vi "test - load and unload.vi"(8 "error in (no error)":errorcluster, 11 "TestCase in":refnum<class "csm-ini-variable-addon.lvclass">) -> (0 "error out":errorcluster, 3 "TestCase out":refnum<class "csm-ini-variable-addon.lvclass">)   [LabVIEW 2017, in "csm-ini-variable-addon.lvclass"]
uses:
  csm-ini-variable-addon.lvclass
  07da2d0f-c6b1-41ab-9bdc-e75734193e5e.vi
  7f30f570-6f21-4deb-b8b3-798b22e0b6ad.vi
  07da2d0f-c6b1-41ab-9bdc-e75734193e5e.vi/b09b9099-6be0-413b-8afc-4908471460c3.vi
  INI-Static-Variable-Support/_Support/FlagInstance-CSMINIVariable.vi
  7f30f570-6f21-4deb-b8b3-798b22e0b6ad.vi/b09b9099-6be0-413b-8afc-4908471460c3.vi
  <userlib>/_NEVSTOP/Communicable State Machine(CSM)/_Support/ChangeFlag/ChangeFlag-Read.vi
  <userlib>/_NEVSTOP/Communicable State Machine(CSM)/_Support/ChangeFlag/ChangeFlagDB.vi
  <vilib>/Utility/Data Type/Get Type Information.vi
  <userlib>/_NEVSTOP/Communicable State Machine(CSM)/addons/API-String-Arugments-Support/_Support/Data To SingleElementsArray_csm.vi
  INI-Static-Variable-Support/_Support/Parse Used Session and Name.vi
  <userlib>/_NEVSTOP/Communicable State Machine(CSM)/addons/API-String-Arugments-Support/_Support/Data To API String Arguments.vi
  INI-Static-Variable-Support/_Support/INI-FGV(lvlibp).vi
  INI-Static-Variable-Support/_Support/Populate String with INI Variable.vi
  <userlib>/_NEVSTOP/Communicable State Machine(CSM)/addons/API-String-Arugments-Support/_Support/Convert API String Arguments to Data(variant).vi
  <userlib>/_NEVSTOP/Communicable State Machine(CSM)/addons/API-String-Arugments-Support/_Support/SingleElementsArray To Data_csm.vi
  <vilib>/addons/_JKI Toolkits/VI Tester/TestCase.llb/TestCase.lvclass
  INI-Static-Variable-Support/INI-Static-Variable-Support.lvlib
  <userlib>/_NEVSTOP/Communicable State Machine(CSM)/addons/API-String-Arugments-Support/API String Arguments Support.lvlib
  C:/Program Files (x86)/National Instruments/LabVIEW 2017/vi.lib/addons/_JKI Toolkits/VI Tester/TestCase.llb/TestCase.lvclass
panel:
  out "String out":string
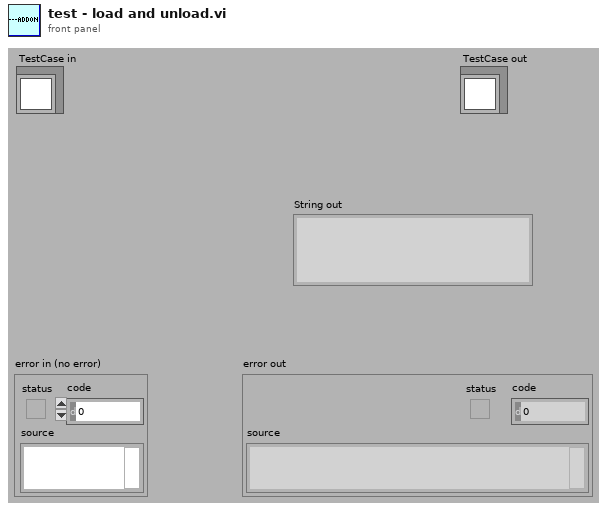
[diagram p1: front panel]
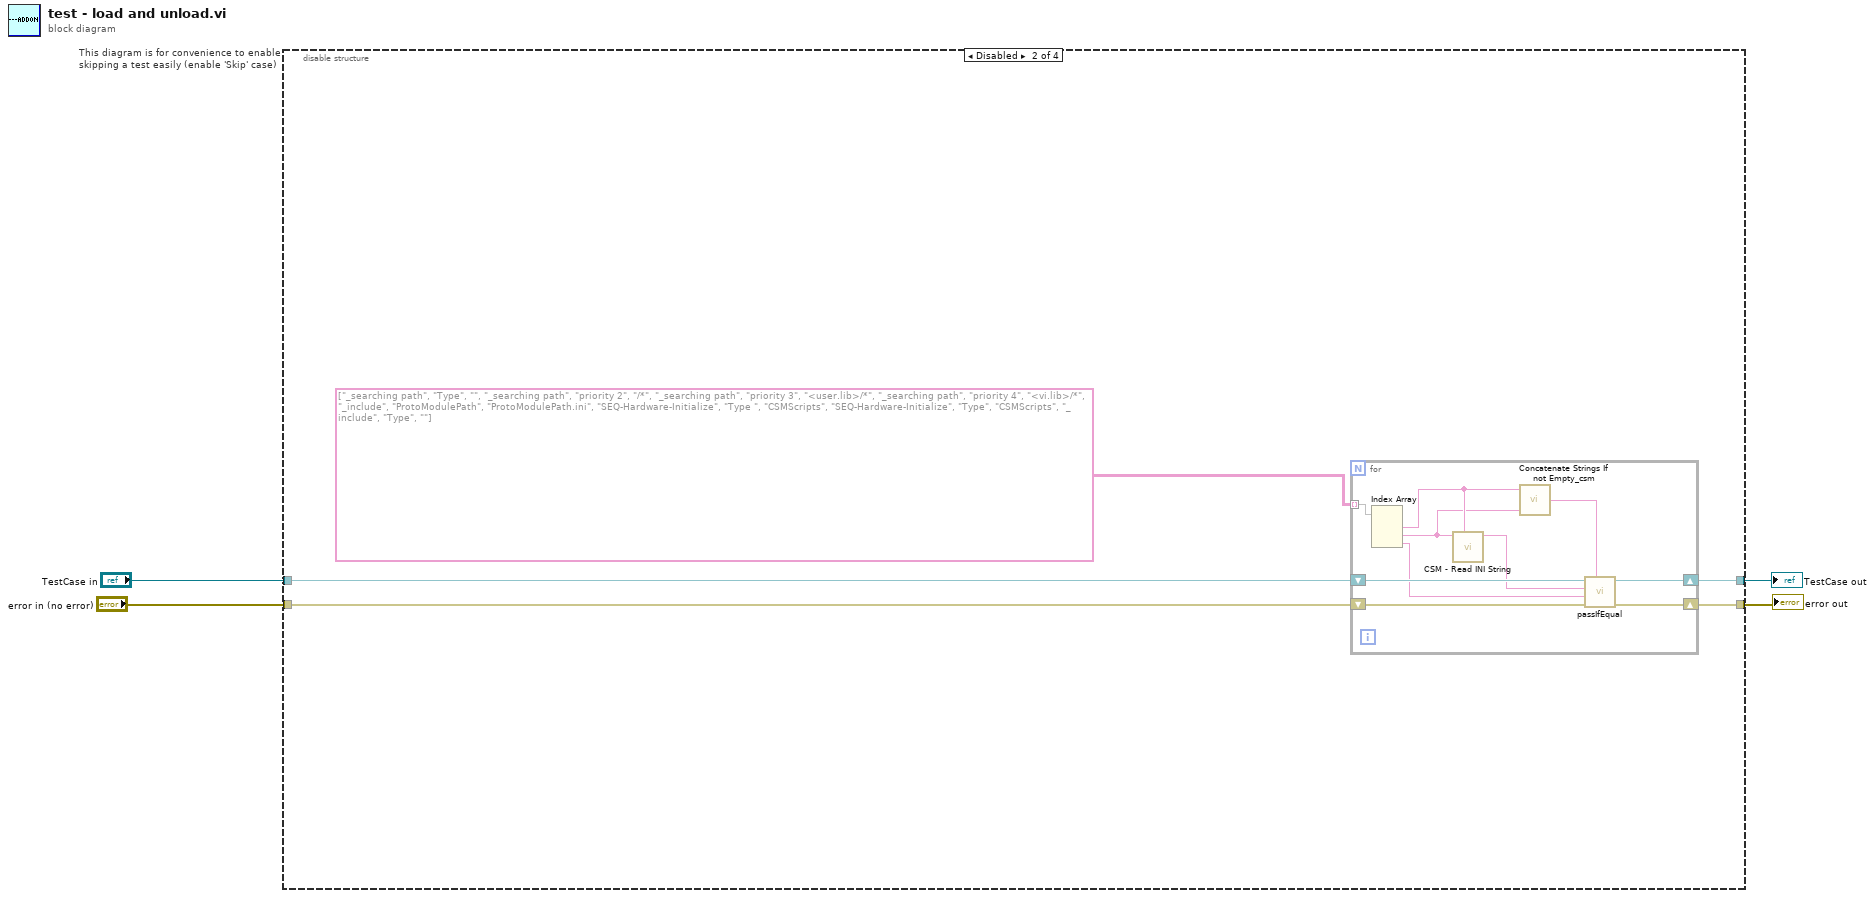
[diagram p0: block diagram]
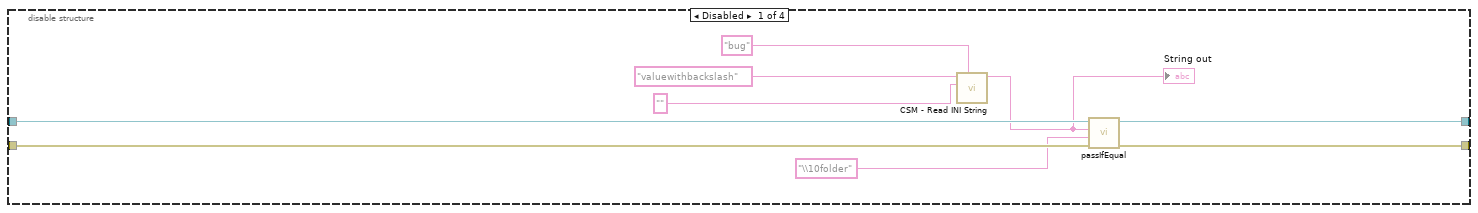
[diagram p2: hidden frame]
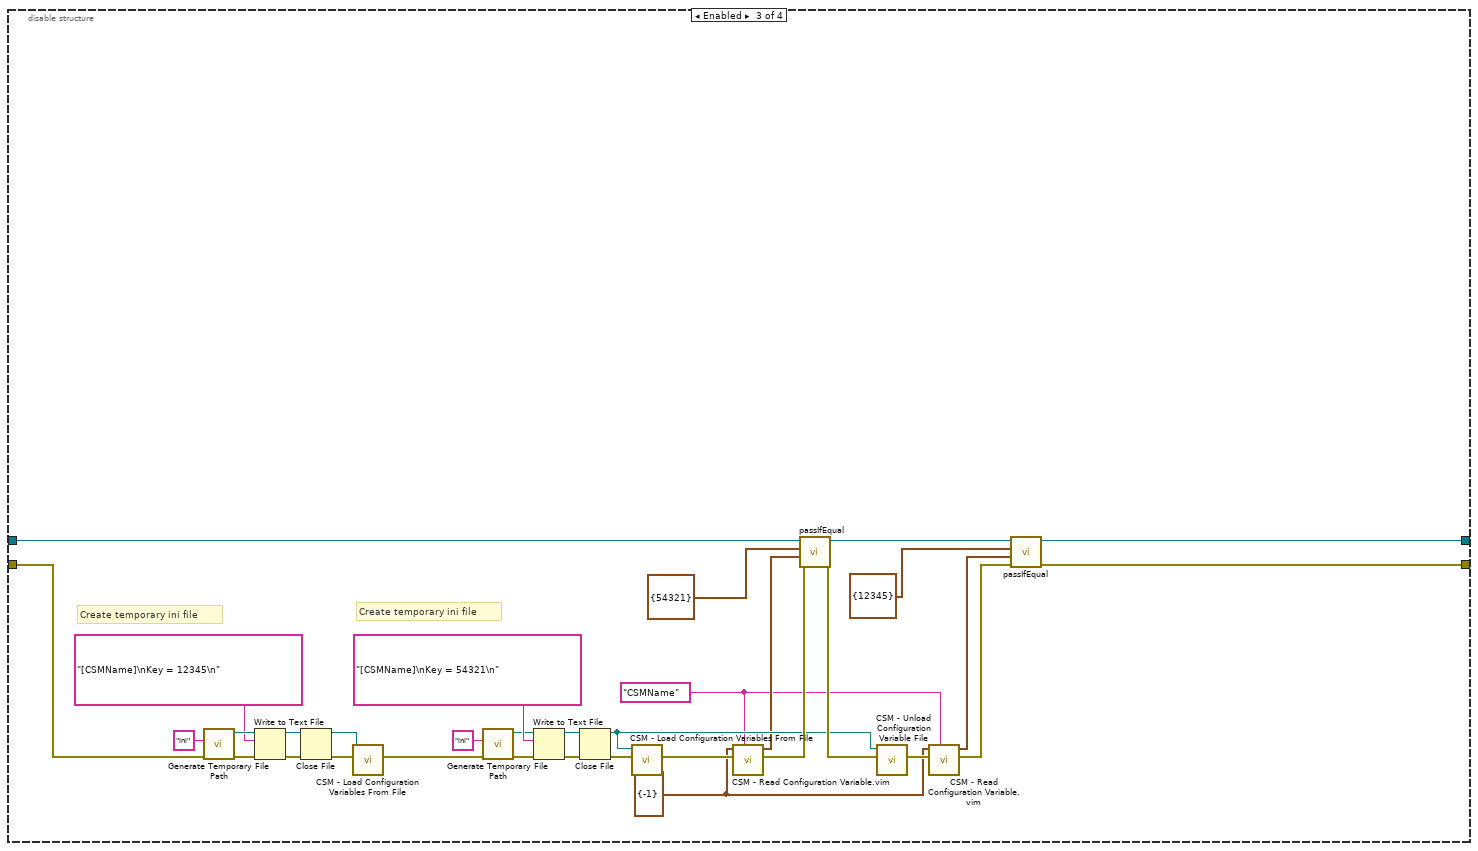
[diagram p3: hidden frame]
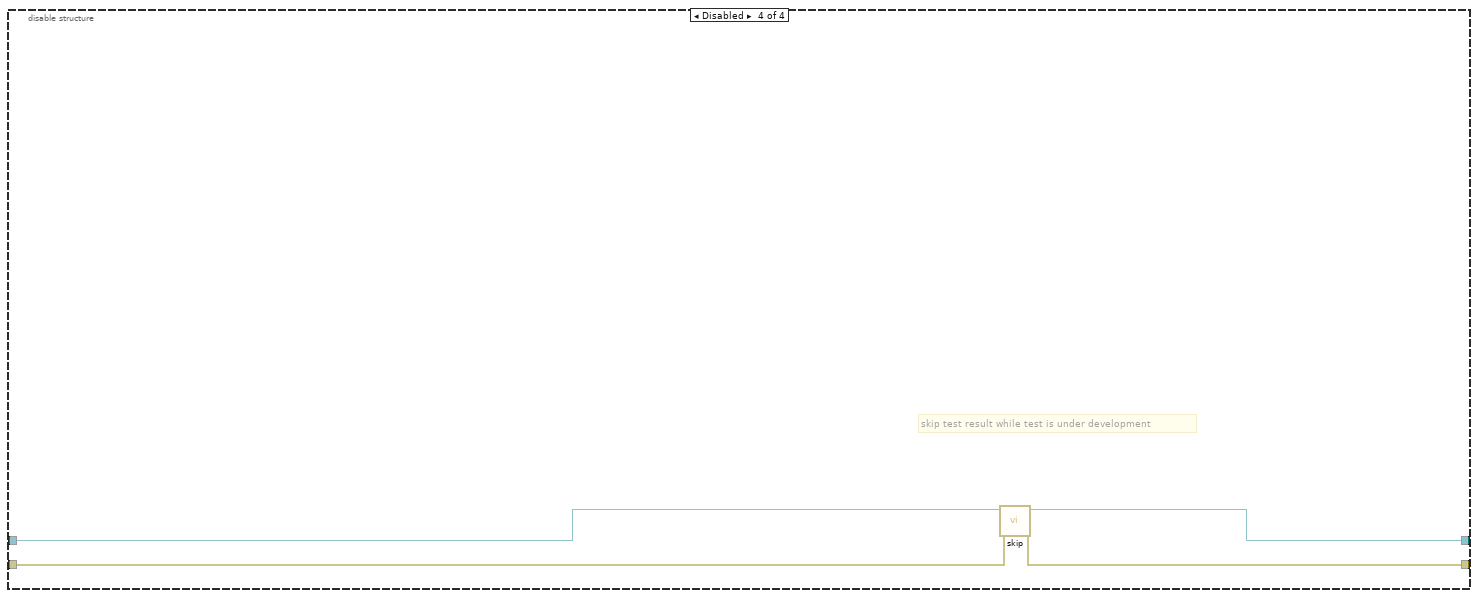
[diagram p4: hidden frame]
diagram:
  n1 = disable-structure "This diagram is for convenience to enable skipping a test easily (enable 'Skip' case)" shown="Disabled" {
    disable-tunnel: "TestCase in" -> [w10 w15 w42 w65]
    disable-tunnel: [w13 w18 w32 w63] -> w1
    disable-tunnel: [w12 w17 w30 w64] -> w3
    disable-tunnel: "error in (no error)" -> [w11 w16 w53 w62]
    frame Disabled {
      n2 = call "CSM - Read INI String.vi"("Section Name(\"\" as Default)"="bug" ("Section Name(\"\" as Default)"), ">> Default Value >>"="" ("String in"), "String in"="valuewithbackslash") -> ("String out"=w6:string)  [unwired: 4 in, 2 out]
      "String out" <- w6
      n3 = call-dynamic "passIfEqual.vi"("error in (no error)"=w11, "y"="\\10folder" ("String in"), "x"=w6, "TestCase in"=w10) -> ("error out"=w12:errorcluster, "TestCase out"=w13:refnum<class "csm-ini-variable-addon.lvclass">)  [unwired: 6 in]
    }
    frame Disabled {
      n4 = for {
        shift-right: [w27] -> w17
        shift-left: w16 -> [w26]
        shift-right: [w28] -> w18
        shift-left: w15 -> [w25]
        tunnel: string[][] [["_searching path", "Type", ""], ["_searching path", "priority 2", "/*"], ["_searching path", "priority 3", "<user.lib>/*"], ["_searching path", "priority 4", "<vi.lib>/*"], ["_include", "ProtoModulePath", "ProtoModulePath.ini"], ["SEQ-Hardware-Initialize", "Type ", "CSMScripts"], ["SEQ-Hardware-Initialize", "Type", "CSMScripts"], ["_include", "Type", ""]] -> [w23] mode=indexing
        n5 = Index Array(array=w23) -> (element #1=w20:string, element #2=w19:string, element #3=w22:string)  [unwired: 3 in]
        n6 = call "CSM - Read INI String.vi"("Section Name(\"\" as Default)"=w20, "String in"=w19) -> ("String out"=w24:string)  [unwired: 5 in, 2 out]
        n7 = call <userlib>:"Concatenate Strings If not Empty_csm.vi"("String"=w19, "prefix"=w20) -> ("result"=w21:string)  [unwired: 3 in]
        n8 = call-dynamic "passIfEqual.vi"("custom report message (\"\")"=w21, "error in (no error)"=w26, "y"=w22, "x"=w24, "TestCase in"=w25) -> ("error out"=w27:errorcluster, "TestCase out"=w28:refnum<class "csm-ini-variable-addon.lvclass">)  [unwired: 5 in]
      }
    }
    frame Enabled {
      w36 = cluster{"Key":i32} {"Key"=-1}
      w29 = "CSMName" ("Section Name(\"\" as Default)")
      # "Create temporary ini file"
      # "Create temporary ini file"
      n9 = call <vilib>:"Generate Temporary File Path.vi"("error in (no error)"=w53, "Temporary File Extension (tmp)"="ini") -> ("error out"=w61:errorcluster, "Unique Temporary File Path"=w58:path)  [unwired: 8 in]
      n10 = Write to Text File(file (use dialog)=w58, text="[CSMName]\nKey = 12345\n", error in=w61) -> (refnum out=w57:refnum<file>, error out=w59:errorcluster)  [unwired: 1 in, 1 out]
      n11 = Close File(refnum=w57, error in=w59) -> (path=w54:path, error out=w56:errorcluster)
      n12 = call "CSM - Load Configuration Variables From File.vi"("error in (no error)"=w56, "Path"=w54) -> ("error out"=w45:errorcluster)  [unwired: 7 in]
      n13 = call <vilib>:"Generate Temporary File Path.vi"("error in (no error)"=w45, "Temporary File Extension (tmp)"="ini") -> ("error out"=w46:errorcluster, "Unique Temporary File Path"=w49:path)  [unwired: 8 in]
      n14 = Write to Text File(file (use dialog)=w49, text="[CSMName]\nKey = 54321\n", error in=w46) -> (refnum out=w50:refnum<file>, error out=w48:errorcluster)  [unwired: 1 in, 1 out]
      n15 = Close File(refnum=w50, error in=w48) -> (path=w40:path, error out=w51:errorcluster)
      n16 = call "CSM - Load Configuration Variables From File.vi"("error in (no error)"=w51, "Path"=w40) -> ("error out"=w44:errorcluster)  [unwired: 7 in]
      n17 = call "CSM - Read Configuration Variable.vim"("Section Name(\"\" as Default)"=w29, "error in (no error)"=w44, "config prototype(Cluster Prefered)"=w36) -> ("error out"=w43:errorcluster, "config out"=w38:cluster{"Key":i32})  [unwired: 5 in]
      n18 = call-dynamic "passIfEqual.vi"("error in (no error)"=w43, "y"=w38, "x"=cluster{"Key":i32} {"Key"=54321}, "TestCase in"=w42) -> ("error out"=w41:errorcluster, "TestCase out"=w35:refnum<class "csm-ini-variable-addon.lvclass">)  [unwired: 6 in]
      n19 = call "CSM - Unload Configuration Variable File.vi"("error in (no error)"=w41, "Path"=w40) -> ("error out"=w37:errorcluster)  [unwired: 7 in]
      n20 = call "CSM - Read Configuration Variable.vim"("Section Name(\"\" as Default)"=w29, "error in (no error)"=w37, "config prototype(Cluster Prefered)"=w36) -> ("error out"=w31:errorcluster, "config out"=w34:cluster{"Key":i32})  [unwired: 5 in]
      n21 = call-dynamic "passIfEqual.vi"("error in (no error)"=w31, "y"=w34, "x"=cluster{"Key":i32} {"Key"=12345}, "TestCase in"=w35) -> ("error out"=w30:errorcluster, "TestCase out"=w32:refnum<class "csm-ini-variable-addon.lvclass">)  [unwired: 6 in]
    }
    frame Disabled {
      # "skip test result while test is under development"
      n22 = call <vilib>:"skip.vi"("error in (no error)"=w62, "TestCase in"=w65) -> ("error out"=w64:errorcluster, "TestCase out"=w63:refnum<class "csm-ini-variable-addon.lvclass">)  [unwired: 8 in]
    }
  }
  "error out" <- w3
  "TestCase out" <- w1
